vi "Mathematics_PiezoVtoZ.vi"(5 "Piezo Amp (21.5)":dbl=21.5, 7 "Piezo Sensitivity (1.95) / nm V-1":dbl=1.95, 8 "Error In":errorcluster, 11 "Piezo Signal In (0) / V":dbl) -> (0 "Error Out":errorcluster, 3 "Piezo Signal Out / nm":dbl)   [LabVIEW 2023]
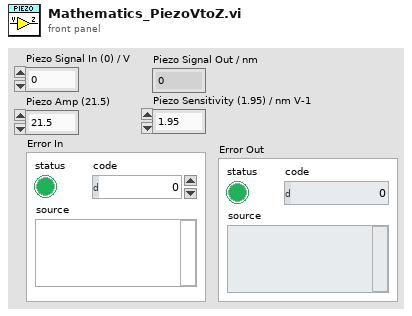
[diagram p1: front panel]
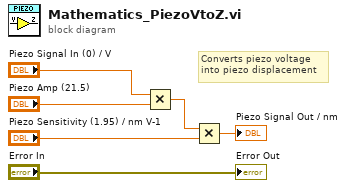
[diagram p0: block diagram]
diagram:
  # "Converts piezo voltage\ninto piezo displacement"
  n1 = Multiply(x="Piezo Signal In (0) / V", y="Piezo Amp (21.5)") -> (x*y=w4:dbl)
  n2 = Multiply(x=w4, y="Piezo Sensitivity (1.95) / nm V-1") -> (x*y=→"Piezo Signal Out / nm":dbl)
  "Error Out" <- "Error In"
